vi "RSZVB Get Pulse Time Start.vi"(8 "error in (no error)":errorcluster {"code" format="%.0x"}, 10 "Channel (1)":i32=1, 11 "VISA session":refnum<visa-resource-name>) -> (0 "error out":errorcluster {"code" format="%.0x"}, 1 "Time Start":dbl format="%^.3e", 3 "dup VISA session":refnum<visa-resource-name>)   [LabVIEW 2011]
doc: "This VI gets the start time of the displayed time range relative to the trigger time.\n\nRemote-control command(s):\n[SENSe<Ch>:]PULSe:TIME:STARt?"
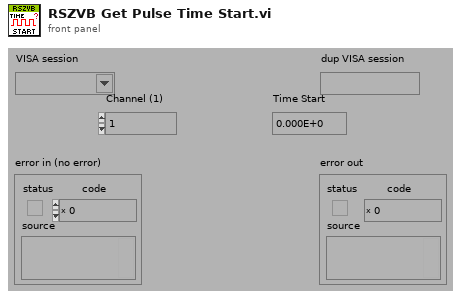
[diagram p1: front panel]
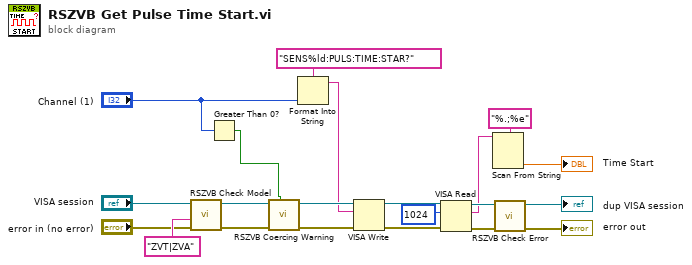
[diagram p0: block diagram]
diagram:
  n1 = call "RSZVB Check Model.vi"("error in (no error)"="error in (no error)", "Model"="ZVT|ZVA" ("Options"), "VISA session"="VISA session") -> ("error out"=w17:errorcluster, "dup VISA session"=w16:refnum<visa-resource-name>)  [unwired: 7 in]
  n2 = Greater Than 0?(x="Channel (1)") -> (x > 0?=w14:bool)
  n3 = call "RSZVB Coercing Warning.vi"("In Range?"=w14, "error in (no error)"=w17, "VISA session"=w16) -> ("error out"=w19:errorcluster, "dup VISA session"=w20:refnum<visa-resource-name>)  [unwired: 7 in]
  n4 = Format Into String(format string="SENS%ld:PULS:TIME:STAR?", "Channel (1)") -> (resulting string=w18:string)  [unwired: 2 in, 1 out]
  n5 = VISA Write(VISA resource name=w20, write buffer=w18, error in (no error)=w19) -> (VISA resource name out=w1:refnum<visa-resource-name>, error out=w2:errorcluster)  [unwired: 1 out]
  n6 = VISA Read(VISA resource name=w1, byte count=u32 1024 ("byte count (0)"), error in (no error)=w2) -> (VISA resource name out=w9:refnum<visa-resource-name>, read buffer=w6:string, error out=w8:errorcluster)  [unwired: 1 out]
  n7 = Scan From String(format string="%.;%e", input string=w6) -> (output 1=→"Time Start":dbl)  [unwired: 3 in, 3 out]
  n8 = call "RSZVB Check Error.vi"("error in (no error)"=w8, "VISA session"=w9) -> ("error out"=→"error out":errorcluster, "dup VISA session"=→"dup VISA session":refnum<visa-resource-name>)  [unwired: 8 in]
